vi "qFSS.vi"(0 "System no.":i32=1 min=1 max=4 step=1, 5 "error in":errorcluster) -> (14 "Scan successful?":bool, 19 "error out":errorcluster)   [LabVIEW 2026]
doc: "Returns the result of the last scan algorithm.\n\nC-887, F-206, M-8X0: Only for GCS syntax version = GCS 2.0 or higher (check with CSV?.vi. If CSV?.vi is not supported, syntax version is GCS 1.0)."
panel:
  # "Returns result of last scan routine."
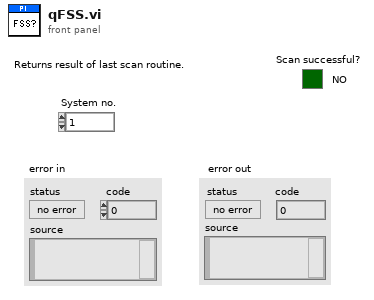
[diagram p1: front panel]
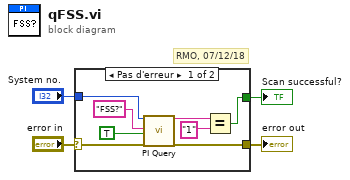
[diagram p0: block diagram]
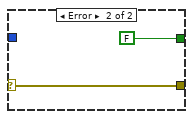
[diagram p2: hidden frame]
diagram:
  # "RMO, 07/12/18"
  n1 = case shown="Pas d'erreur" "error in" {
    selector: "error in" -> [w5 w14]
    tunnel: "System no." -> [w11 _]
    tunnel: [w9 FALSE] -> w3
    tunnel: [w7 w14] -> w2
    frame No Error {
      n2 = call "PI Query.vi"("System no."=w11, "String to send"="FSS?", "Attach termination char.?"=TRUE ("Attach Linefeed?"), "error in"=w5) -> ("String read"=w6:string, "error out"=w7:errorcluster)  [unwired: 3 in, 11 out]
      n3 = Equal?(x=w6, y="1") -> (x = y?=w9:bool)
    }
    frame Error {
    }
  }
  "error out" <- w2
  "Scan successful?" <- w3
